vi "Menu Act PNG Json Gen.vi"(8 "error in (no error)":errorcluster, 11 "Main Panel in":refnum<class "Main Panel.lvclass">) -> (0 "error out":errorcluster, 3 "Main Panel out":refnum<class "Main Panel.lvclass">)   [LabVIEW 2018, in "Main Panel.lvlib" / "Main Panel.lvclass"]
uses:
  Main Panel.lvclass
  C:/Program Files (x86)/National Instruments/LabVIEW 2018/vi.lib/MGI/Panel Manager/Panel Actor/Panel Actor/Panel Actor.lvclass
  Pic Json Generator/Pic Json Generator/Pic Json Generator.lvclass
  Main Panel.lvclass/Main Panel.ctl
  <vilib>/MGI/Panel Manager/Panel/Panel/Window/Window.lvclass
  C:/Program Files (x86)/National Instruments/LabVIEW 2018/vi.lib/MGI/Panel Manager/Panel/Panel/Panel.lvclass
  <vilib>/MGI/Panel Manager/Panel/Panel/Window/Window.vi
  <vilib>/MGI/Panel Manager/Panel Actor/Panel Actor/Panel Actor.lvclass
  <vilib>/MGI/Panel Manager/Panel/Panel.lvlib
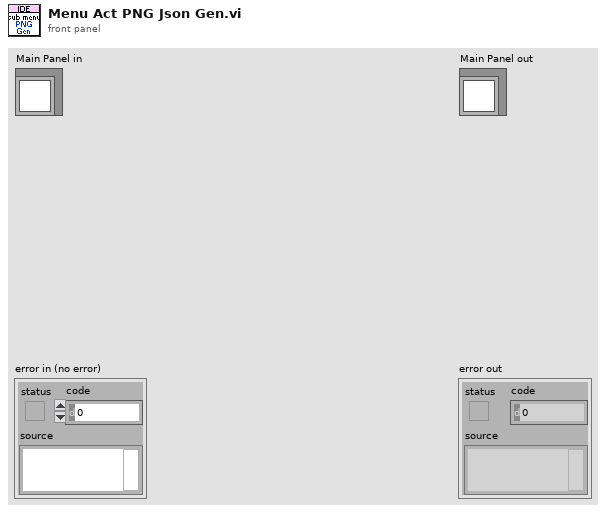
[diagram p1: front panel]
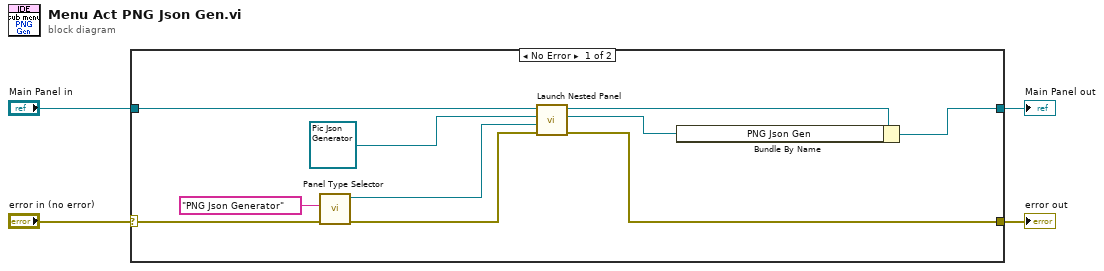
[diagram p0: block diagram]
diagram:
  n1 = case shown="No Error" "error in (no error)" {
    selector: "error in (no error)" -> [w6 w16]
    tunnel: [w5 w16] -> w3
    tunnel: [w9 w15] -> w1
    tunnel: "Main Panel in" -> [w10 w15]
    frame No Error {
      n2 = call-poly <vilib>:"Panel Type Selector.vi"("error in (no error)"=w6, "Default Title"="PNG Json Generator") -> ("error out"=w12:errorcluster, "Window out"=w13:refnum<class "Window.lvclass">)  [unwired: 8 in]
      n3 = call <vilib>:"Launch Nested Panel.vi"("error in (no error)"=w12, "Panel"=w13, "Nested Panel Actor"=refnum<class "Pic Json Generator.lvclass"> refnum ("Pic Json Generator.lvlib:Pic Json Generator.lvclass"), "Panel Actor in"=w10) -> ("error out"=w5:errorcluster, "Nested Actor's Enqueuer"=w7:refnum<class "Message Enqueuer.lvclass">, "Panel Actor out"=w8:refnum<class "Main Panel.lvclass">)  [unwired: 4 in, 1 out]
      n4 = Bundle By Name(cluster=w8, "PNG Json Gen"=w7) -> (w9:refnum<class "Main Panel.lvclass">)
    }
    frame Error {
    }
  }
  "error out" <- w3
  "Main Panel out" <- w1
